vi "Publish Reading.vi"(8 "error in (no error)":errorcluster, 11 "CS++DMM in":refnum<class "CS++DMM.lvclass">) -> (0 "error out":errorcluster, 3 "CS++DMM out":refnum<class "CS++DMM.lvclass">)   [LabVIEW 2013, in "CS++DMM.lvlib" / "CS++DMM.lvclass"]
doc: "Publish Reading to PV."
uses:
  CS++DMM.lvclass
  CSPP_Core/Classes/CS++ProcessVariables/ProcessVariable/PV.lvclass
  CS++DMM.lvclass/CS++DMM.ctl
  CSPP_Core/Classes/CS++ProcessVariables/PVConnection/PVConnection.lvclass
  CSPP_Core/Classes/CS++ProcessVariables/ProcessVariable/PV.lvclass/PV.ctl
  CSPP_Core/Classes/CS++ProcessVariables/ProcessVariable/Write Data.vi
  CSPP_Core/Classes/CS++ProcessVariables/ProcessVariable/Write Timestamp.vi
  CSPP_Core/Classes/CS++ProcessVariables/ProcessVariable/Write Quality.vi
  CSPP_Core/Classes/CS++ProcessVariables/ProcessVariable/Write status.vi
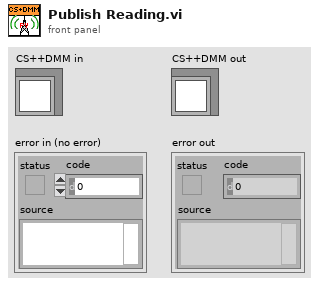
[diagram p1: front panel]
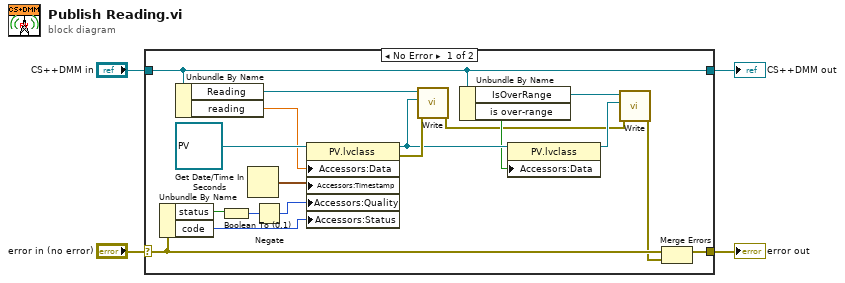
[diagram p0: block diagram]
diagram:
  n1 = case shown="No Error" "error in (no error)" {
    selector: "error in (no error)" -> [w14 w24]
    tunnel: [w13 w24] -> w3
    tunnel: [w12 w23] -> w1
    tunnel: "CS++DMM in" -> [w12 w23]
    frame No Error {
      n2 = Unbundle By Name(w14) -> ("status"=w19:bool, "code"=w16:i32)
      n3 = Unbundle By Name(w12) -> ("Reading"=w22:refnum<class "PVConnection.lvclass">, "reading"=w20:dbl)
      n4 = Boolean To (0,1)(Boolean=w19) -> (0, 1=w18:i16)
      n5 = Get Date/Time In Seconds() -> (seconds since 1Jan1904=w8:timestamp)
      n6 = Negate(x=w18) -> (-x=w17:i16)
      n7 = property class="PV.lvclass"(reference=refnum<class "PV.lvclass"> refnum ("CS++ProcessVariables.lvlib:PV.lvclass"), "Accessors:Data"=w20, "Accessors:Timestamp"=w8, "Accessors:Quality"=w17, "Accessors:Status"=w16) -> (reference out=w10:refnum<class "PV.lvclass">, error out=w15:errorcluster)  [unwired: 1 in]
      n8 = call-dynamic "Write.vi"("error in (no error)"=w15, "PV"=w10, "PVConnection in"=w22) -> ("error out"=w6:errorcluster)  [unwired: 7 in, 1 out]
      n9 = Unbundle By Name(w12) -> ("IsOverRange"=w11:refnum<class "PVConnection.lvclass">, "is over-range"=w9:bool)
      n10 = property class="PV.lvclass"(reference=w10, "Accessors:Data"=w9) -> (reference out=w7:refnum<class "PV.lvclass">)  [unwired: 1 in, 1 out]
      n11 = call-dynamic "Write.vi"("error in (no error)"=w6, "PV"=w7, "PVConnection in"=w11) -> ("error out"=w5:errorcluster)  [unwired: 7 in, 1 out]
      n12 = Merge Errors(w14, w5) -> (w13:errorcluster)
    }
    frame Error {
    }
  }
  "error out" <- w3
  "CS++DMM out" <- w1
